vi "ADC settings.vi"(8 "Error In":errorcluster, 10 "ADC settings in":T1={"ADCspeed"=1.0, "ADCgain"=1.0, "ADC Integrate"=1.0, "sampling \nfrequency (Hz)"=1.0}, 11 "mode (R)":enum16{"read", "write"}(ring)=enum."write") -> (0 "Error out":errorcluster, 2 "ADC settings out":T1={"ADCspeed"=1.0, "ADCgain"=1.0, "ADC Integrate"=1.0, "sampling \nfrequency (Hz)"=1.0})   [LabVIEW 2014]
doc: "Functional Global Variable for the algorithm settings. The used method as well as the max. Iteration steps and the tolerance can be given. In addition, the algorithm can be told to use boundaries (if possible)."
uses:
  controls/ADC settings.ctl
panel:
  # "Input"
  # "Output"
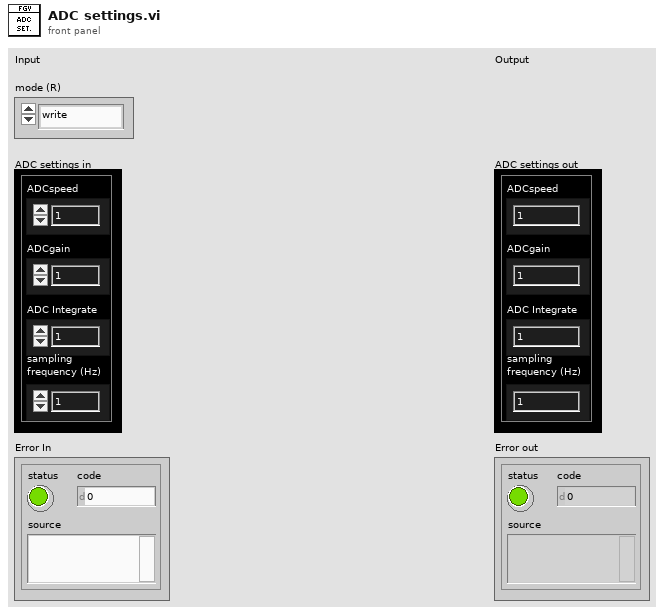
[diagram p1: front panel]
types:
  T1 = typedef "ADC settings.ctl" = cluster{"ADCspeed":dbl, "ADCgain":dbl, "ADC Integrate":dbl, "sampling \nfrequency (Hz)":dbl}
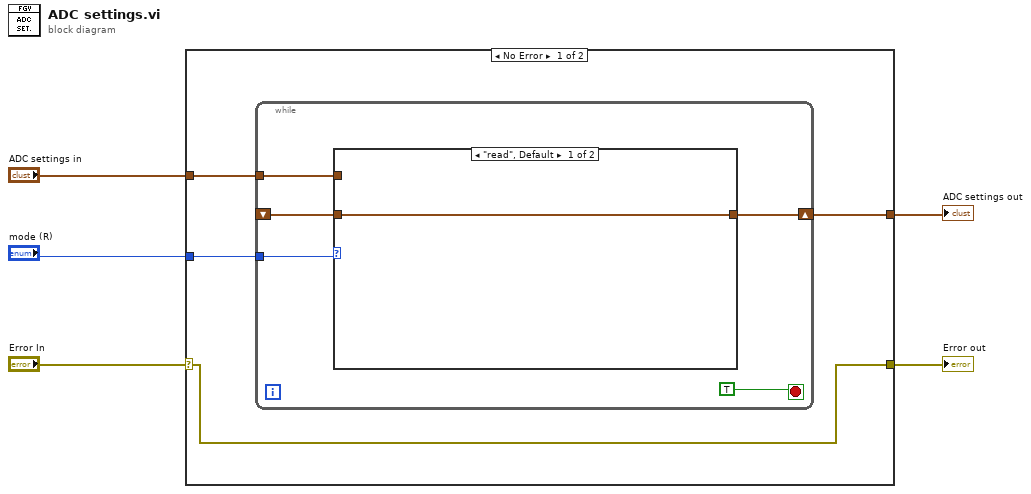
[diagram p0: block diagram]
diagram:
  n1 = case shown="No Error" "Error In" {
    selector: "Error In" -> [w6 w18]
    tunnel: "mode (R)" -> [w9 _]
    tunnel: [w6 w18] -> w4
    tunnel: "ADC settings in" -> [w8 w17]
    tunnel: [w7 w17] -> w2
    frame No Error {
      n2 = while {
        tunnel: w9 -> [w13]
        tunnel: w8 -> [w12]
        shift-right: [w10] -> w7
        shift-left: _ -> [w11]
        stop <- TRUE stop-if-true
        n3 = case shown="\"read\", Default" w13 {
          tunnel: w12 -> [_ w16]
          tunnel: w11 -> [w15 _]
          tunnel: [w15 w16] -> w10
          frame "read", Default {
          }
          frame "write" {
          }
        }
      }
    }
    frame Error {
    }
  }
  "Error out" <- w4
  "ADC settings out" <- w2
